vi "练习3-输出连续波形.vi"() -> ()   [LabVIEW 2021]
panel:
  out "Waveform Graph":dynamicdata(graph)
  in  "stop":bool
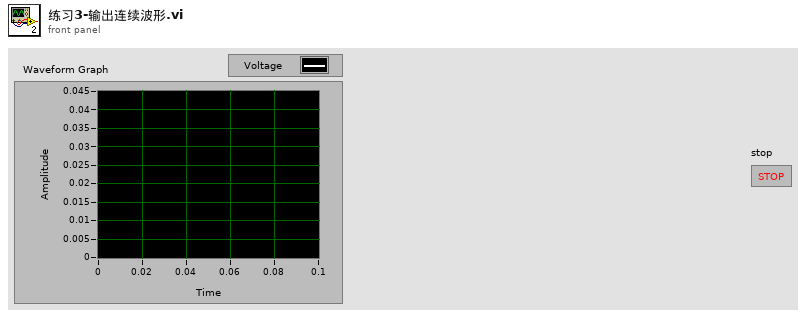
[diagram p1: front panel]
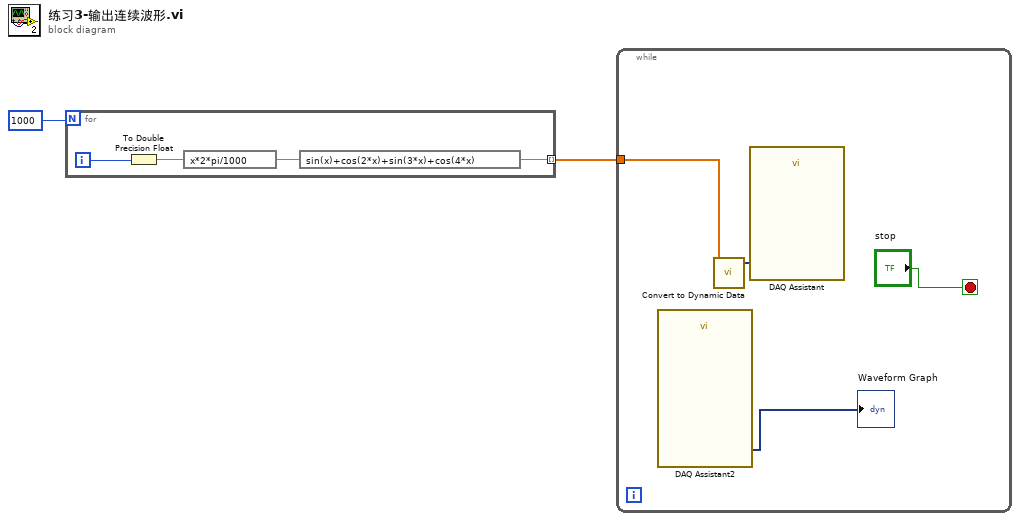
[diagram p0: block diagram]
diagram:
  n1 = for {
    N: 1000 -> [_]
    tunnel: [w3] -> w1 mode=indexing
    i -> [w6]
    n2 = To Double Precision Float(number=w6) -> (double precision float=w5:dbl)
    n3 = expression code="x*2*pi/1000"(w5) -> (w4:dbl)
    n4 = expression code="sin(x)+cos(2*x)+sin(3*x)+cos(4*x)"(w4) -> (w3:dbl)
  }
  n5 = while {
    tunnel: w1 -> [w9]
    stop <- "stop" stop-if-true
    n6 = call "DAQ Assistant2"() -> ("data"=→"Waveform Graph":dynamicdata)  [unwired: 17 in, 2 out]
    n7 = call "Convert to Dynamic Data"("Array"=w9) -> ("Dynamic Data Type"=w8:dynamicdata)  [unwired: 3 in]
    n8 = call "DAQ Assistant"("data"=w8) -> ()  [unwired: 16 in, 3 out]
  }
